vi "Addition.vi"() -> ()   [LabVIEW 2020]
panel:
  out "initialized array 3":bool[](array[boolean])
  out "Sum":dbl
  out "initialized array 2":bool[](array[boolean])
  in  "B":dbl
  out "initialized array":bool[](array[boolean])
  in  "A":dbl
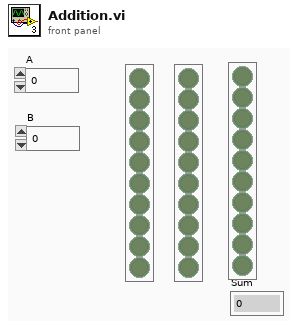
[diagram p1: front panel]
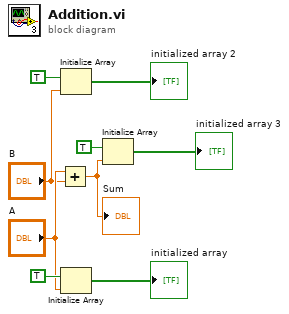
[diagram p0: block diagram]
diagram:
  n1 = Add(x="A", y="B") -> (x+y=w1:dbl)
  "Sum" <- w1
  n2 = Initialize Array "Initialize Array"(TRUE, "B") -> (→"initialized array 2":bool[])
  n3 = Initialize Array "Initialize Array"(TRUE, "A") -> (→"initialized array":bool[])
  n4 = Initialize Array "Initialize Array"(TRUE, w1) -> (→"initialized array 3":bool[])
